vi "Group Page.vi"(8 "error in":errorcluster, 11 "Node Ptr":T1 format="%.0x") -> (0 "error out":errorcluster)   [LabVIEW 2027, in "Embedded Data Logger System Explorer.lvlib"]
uses:
  Embedded Data Logger System Explorer.lvlib
  <vilib>/NI VeriStand/Custom Device API/Custom Device Item Ref.ctl
  <vilib>/NI VeriStand/Custom Device API/Custom Device API.lvlib
panel:
  in  "Header":cluster{"Section Name":string}={"Section Name"=" Settings"}
  in  "Description":string
  out "Name":string
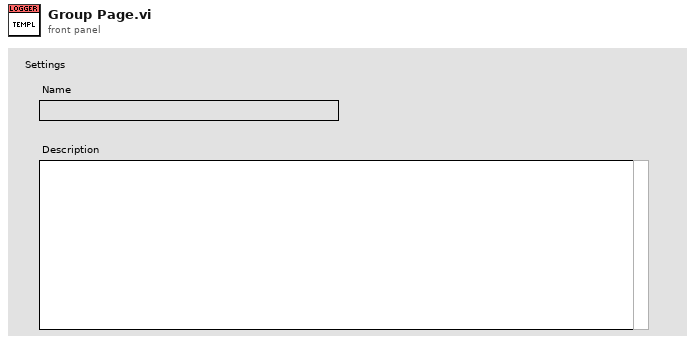
[diagram p1: front panel]
types:
  T1 = typedef "Custom Device API.lvlib/Custom Device Item Ref.ctl" = u64
  T2 = typedef "Custom Device API.lvlib/Custom Device Item Info.ctl" = cluster{"Name":string, "Is Channel":bool, "GUID":string, "Is Waveform":bool}
  T3 = typedef "Custom Device API.lvlib/Custom Device Commands.ctl" = enum16{"Default", "Item renamed", "Shutdown", "Dynamic button pressed"}
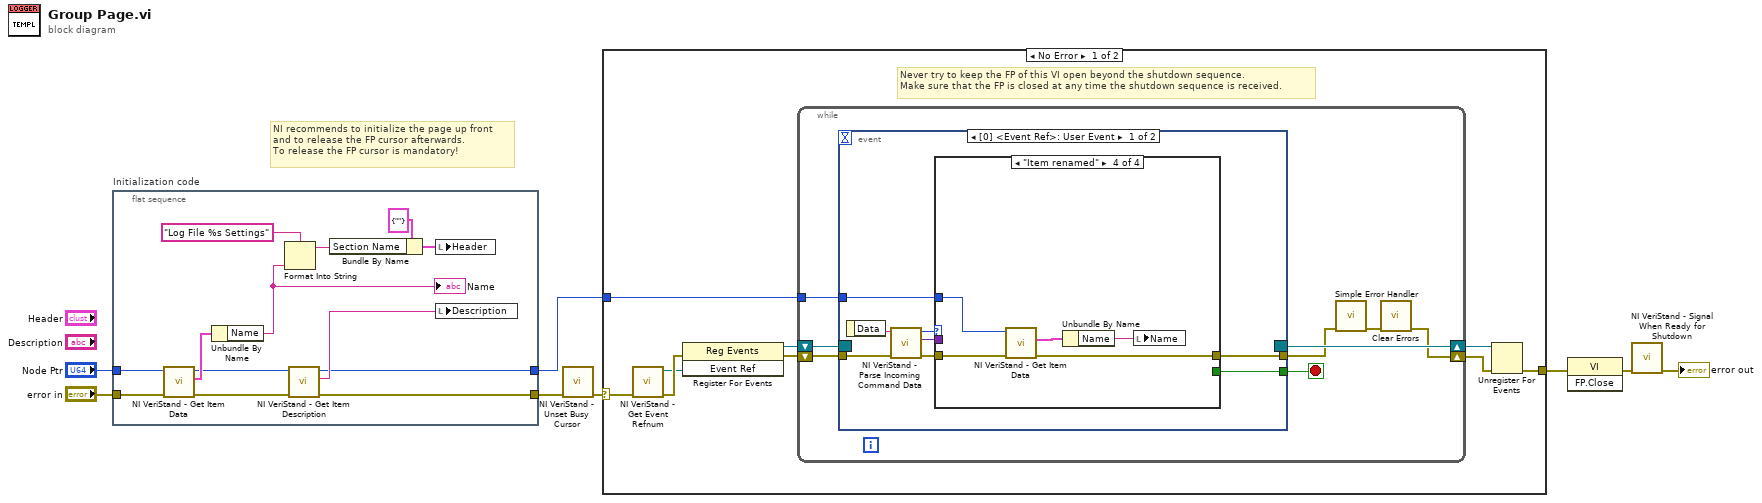
[diagram p0: block diagram]
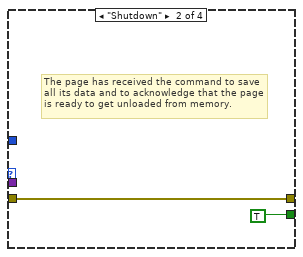
[diagram p3: hidden frame]
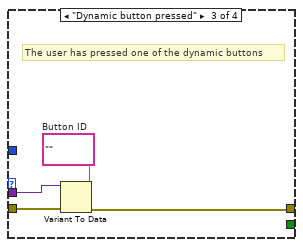
[diagram p4: hidden frame]
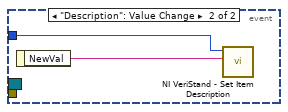
[diagram p5: hidden frame]
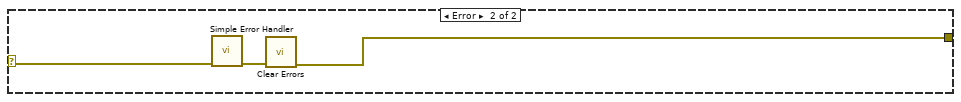
[diagram p6: hidden frame]
diagram:
  # "NI recommends to initialize the page up front\nand to release the FP cursor afterwards.\nTo release the FP cursor is mandatory!"
  n1 = flat-sequence "Initialization code" {
    tunnel: "error in" -> [w11]
    tunnel: "Node Ptr" -> [w10]
    tunnel: [w13] -> w4
    tunnel: [w14] -> w2
    frame #0 {
      n2 = call <vilib>:"NI VeriStand - Get Item Data.vi"("error in (no error)"=w11, "Item Ref in"=w10) -> ("error out"=w12:errorcluster, "Item Info"=w20:T2, "Item Ref out"=w15:T1)  [unwired: 7 out]
      n3 = Unbundle By Name(w20) -> ("Name"=w9:string)
      "Name" <- w9
      n4 = Format Into String(format string="Log File %s Settings" ("Section Name"), w9) -> (resulting string=w17:string)  [unwired: 2 in, 1 out]
      n5 = call <vilib>:"NI VeriStand - Get Item Description.vi"("error in (no error)"=w12, "Item Ref in"=w15) -> ("error out"=w13:errorcluster, "Description"=w21:string, "Item Ref out"=w14:T1)  [unwired: 7 out]
      n6 = Bundle By Name(cluster=cluster{"Section Name":string} {"Section Name"=""} ("header"), "Section Name"=w17) -> (w16:cluster{"Section Name":string})
      n7 = local write "Header"(w16) -> ()
      n8 = local write "Description"(w21) -> ()
    }
  }
  n9 = call <vilib>:"NI VeriStand - Unset Busy Cursor.vi"("error in (no error)"=w4) -> ("error out"=w3:errorcluster)  [unwired: 10 out]
  n10 = case shown="No Error" w3 {
    selector: w3 -> [w23 w63]
    tunnel: [w22 w61] -> w8
    tunnel: w2 -> [w24 _]
    frame No Error {
      # "Never try to keep the FP of this VI open beyond the shutdown sequence.\nMake sure that the FP is closed at any time the shutdown sequence is received."
      n11 = call <vilib>:"NI VeriStand - Get Event Refnum.vi"("error in (no error)"=w23) -> ("error out"=w30:errorcluster, "Event Ref"=w27:refnum<user-event>)  [unwired: 9 out]
      n12 = register-events(error in=w30, w27) -> (reference out=w25:refnum<event-registration>, error out=w26:errorcluster)  [unwired: 1 in]
      n13 = while {
        tunnel: w24 -> [w34]
        shift-right: [w31] -> w28
        shift-left: w26 -> [w37]
        shift-right: [w38] -> w29
        shift-left: w25 -> [w36]
        stop <- w35 stop-if-true
        n14 = event shown="[0] <Event Ref>: User Event" {
          selector: w36 -> [_ _]
          dyn-events: [_ _] -> w38
          timeout: _ -> [_ _]
          tunnel: w37 -> [w46 _]
          tunnel: [w42 _] -> w35
          tunnel: [w41 _] -> w33
          tunnel: w34 -> [w40 w59]
          event User Event {
            n15 = event-data() -> ("Data"=w45:string)  [unwired: 1 out]
            n16 = call <vilib>:"NI VeriStand - Parse Incoming Command Data.vi"("error in (no error)"=w46, "Incoming data"=w45) -> ("error out"=w44:errorcluster, "Outgoing data"=w39:variant, "Action"=w43:T3)  [unwired: 7 out]
            n17 = case shown="\"Item renamed\"" w43 {
              tunnel: w44 -> [w47 w48 w53 w57]
              tunnel: [_ TRUE _ _] -> w42
              tunnel: [w47 w48 w51 w56] -> w41
              tunnel: w40 -> [_ _ _ w55]
              tunnel: w39 -> [_ _ w52 _]
              frame "Default" {
              }
              frame "Shutdown" {
                # "The page has received the command to save all its data and to acknowledge that the page is ready to get unloaded from memory."
              }
              frame "Dynamic button pressed" {
                w50 = ""  # Button ID
                # "The user has pressed one of the dynamic buttons"
                n18 = Variant To Data(error in=w53, type=w50, Variant=w52) -> (error out=w51:errorcluster)  [unwired: 1 out]
              }
              frame "Item renamed" {
                n19 = call <vilib>:"NI VeriStand - Get Item Data.vi"("error in (no error)"=w57, "Item Ref in"=w55) -> ("error out"=w56:errorcluster, "Item Info"=w58:T2)  [unwired: 8 out]
                n20 = Unbundle By Name(w58) -> ("Name"=w54:string)
                n21 = local write "Name"(w54) -> ()
              }
            }
          }
          event "Description": Value Change {
            n22 = event-data() -> ("NewVal"=w60:string)  [unwired: 1 out]
            n23 = call <vilib>:"NI VeriStand - Set Item Description.vi"("Description"=w60, "Item Ref in"=w59) -> ()  [unwired: 1 in, 9 out]
          }
        }
        n24 = call <vilib>:"Simple Error Handler.vi"("error in (no error)"=w33) -> ("error out"=w32:errorcluster)  [unwired: 1 in, 7 out]
        n25 = call <vilib>:"Clear Errors.vi"("error in (no error)"=w32) -> ("error out"=w31:errorcluster)  [unwired: 1 in, 5 out]
      }
      n26 = Unregister For Events(event registration refnum=w29, error in=w28) -> (error out=w22:errorcluster)
    }
    frame Error {
      n27 = call <vilib>:"Simple Error Handler.vi"("error in (no error)"=w63) -> ("error out"=w62:errorcluster)  [unwired: 1 in, 7 out]
      n28 = call <vilib>:"Clear Errors.vi"("error in (no error)"=w62) -> ("error out"=w61:errorcluster)  [unwired: 1 in, 5 out]
    }
  }
  n29 = invoke class="VI" method="FP.Close"(error in=w8) -> (error out=w7:errorcluster)  [unwired: 2 in, 2 out]
  n30 = call <vilib>:"NI VeriStand - Signal When Ready for Shutdown.vi"("error in (no error)"=w7) -> ("error out"=→"error out":errorcluster)  [unwired: 10 out]
